vi "Update DAQ Parameters.vi"(8 "error in (no error)":errorcluster={"status"=FALSE, "code"=0, "source"="Abort\rATS : ApiSuccess (512)"}, 11 "DAQ Class in":refnum<class "DAQ Class.lvclass">=refnum) -> (0 "error out":errorcluster={"status"=FALSE, "code"=0, "source"="Abort\rATS : ApiSuccess (512)"}, 2 "DAQ Parameters Out":T1={"Points Per A-Scan"=1024, "A-Scans Per B-Scan"=250, "Number of B-Scans"=1, "A-Scans Per Transfer"=1, "Trigger Voltage"=0.0, "Trigger Source"=enum."External", "Trigger Slope"=enum."Rising", "Channel"=enum."Channel 1", "Clock"=enum."Internal Clock", "Bits per Sample"=0.0, "Range"=0.0}, 3 "DAQ Class out":refnum<class "DAQ Class.lvclass">)   [LabVIEW 2014, in "DAQ Class.lvclass"]
uses:
  DAQ Class.lvclass
  ATS660/ATS660 Class.lvclass
  DAQ Parameters.ctl
  Trigger Source.ctl
  Trigger Slope.ctl
  Type Defs/OCT DAQ Channel Data Type.ctl
  Clock Control.ctl
panel:
  in  "DAQ Parameters":T1={"Points Per A-Scan"=1280, "A-Scans Per B-Scan"=250, "Number of B-Scans"=1, "A-Scans Per Transfer"=250, "Trigger Voltage"=140.0, "Trigger Source"=enum."External", "Trigger Slope"=enum."Rising", "Channel"=enum."Channel 1", "Clock"=enum."External Clock", "Bits per Sample"=16.0, "Range"=4.0}
  in  "OK Button":bool
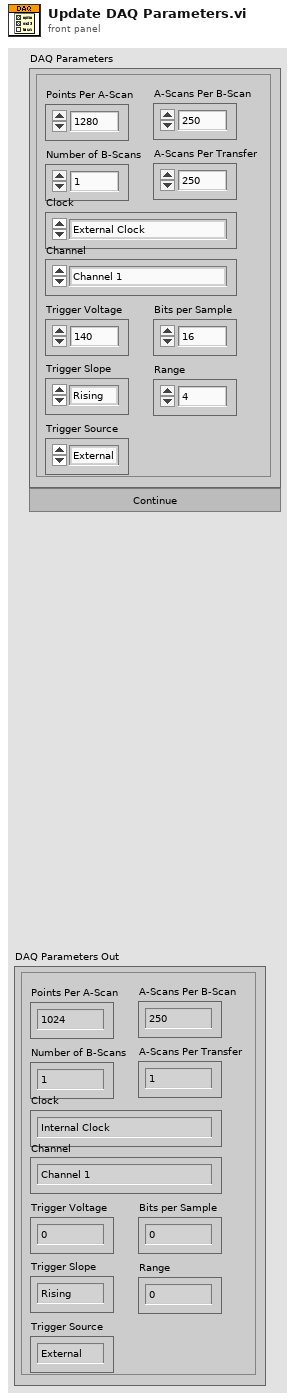
[diagram p1: front panel]
types:
  T1 = typedef "DAQ Class.lvclass/DAQ Parameters.ctl" = cluster{"Points Per A-Scan":u32, "A-Scans Per B-Scan":u32, "Number of B-Scans":u32, "A-Scans Per Transfer":u32, "Trigger Voltage":sgl, "Trigger Source":T2, "Trigger Slope":T3, "Channel":T4, "Clock":T5, "Bits per Sample":dbl, "Range":dbl}
  T2 = typedef "DAQ Class.lvclass/Trigger Source.ctl" = enum16{"External", "Channel A", "Channel B"}
  T3 = typedef "DAQ Class.lvclass/Trigger Slope.ctl" = enum16{"Rising", "Falling"}
  T4 = typedef "OCT DAQ Channel Data Type.ctl" = enum16{"Channel 1", "Channel 2", "Channel 1 and 2"}
  T5 = typedef "DAQ Class.lvclass/Clock Control.ctl" = enum16{"Internal Clock", "External Clock"}
  T6 = enum8{"Enabled", "Disabled", "Disabled and Grayed Out"}
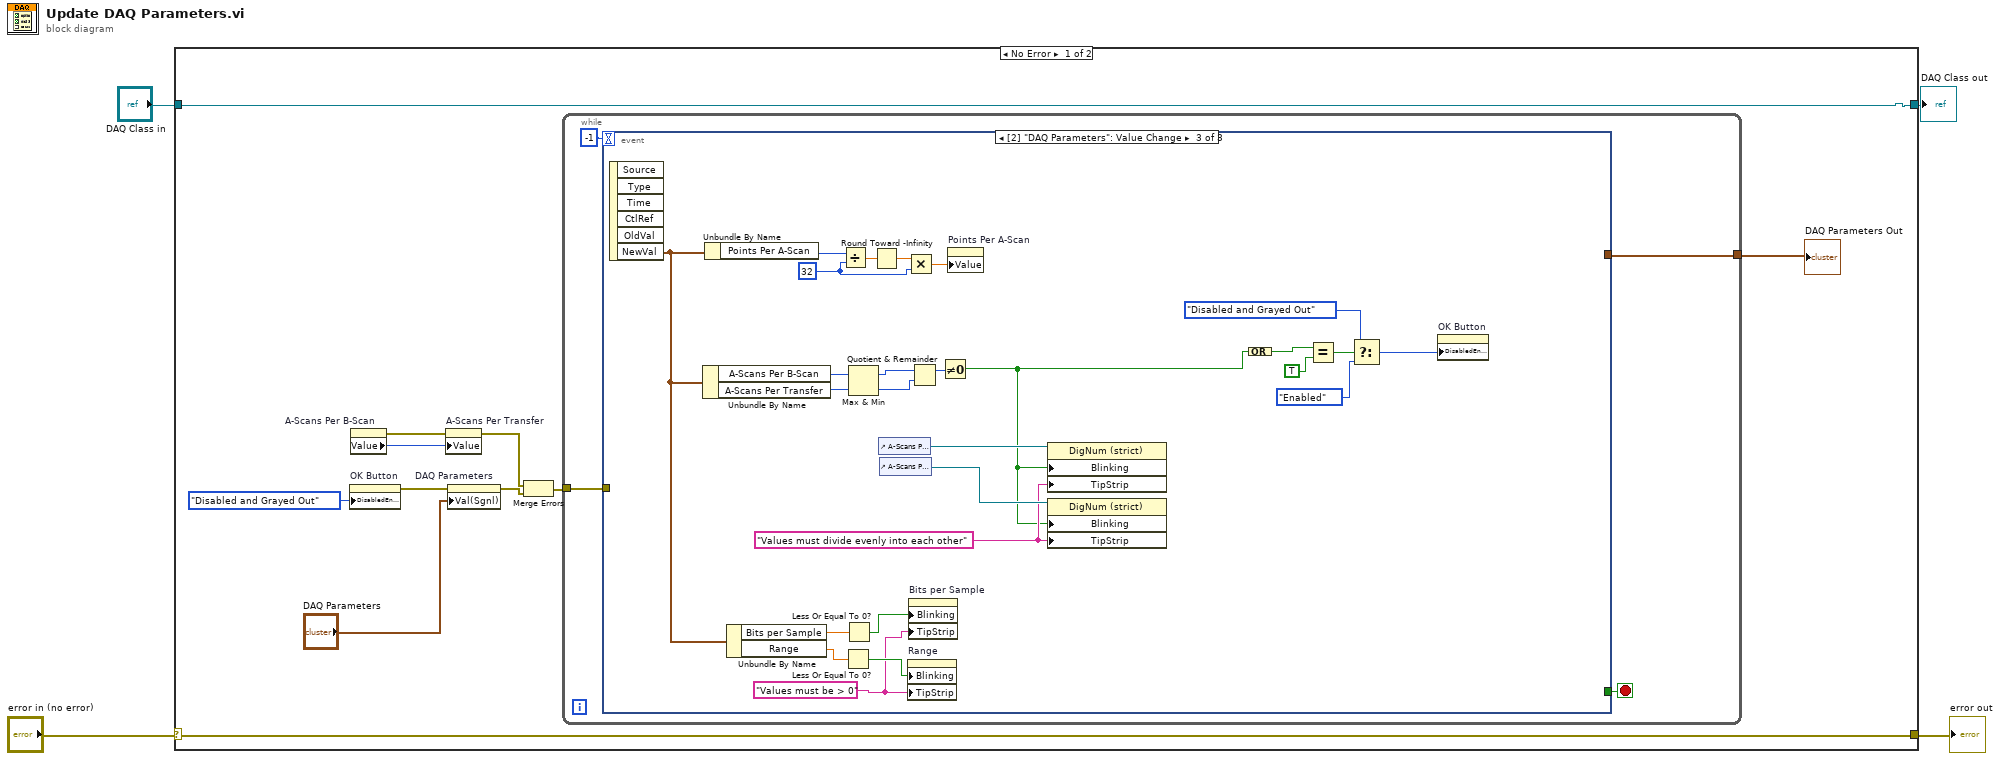
[diagram p0: block diagram]
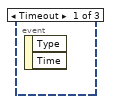
[diagram p2: hidden frame]
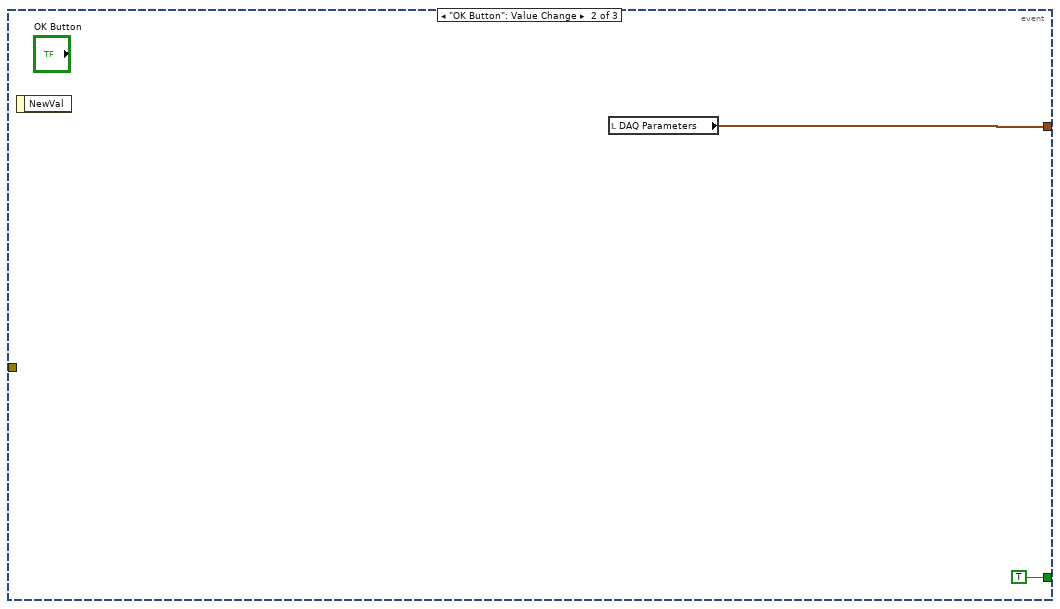
[diagram p3: hidden frame]
diagram:
  n1 = case shown="No Error" "error in (no error)" {
    selector: "error in (no error)" -> [w15 w49]
    tunnel: [w15 w49] -> w3
    tunnel: [w14 w48] -> w1
    tunnel: "DAQ Class in" -> [w14 w48]
    frame No Error {
      n2 = property on="OK Button" class="Bool"("DisabledEnum"=T6."Disabled and Grayed Out" ("Disabled")) -> (error out=w11:errorcluster)  [unwired: 2 in, 1 out]
      n3 = property on="A-Scans Per B-Scan" class="DigNum (strict)"() -> (error out=w10:errorcluster, "Value"=w9:u32)  [unwired: 2 in, 1 out]
      n4 = property on="A-Scans Per Transfer" class="DigNum (strict)"(error in=w10, "Value"=w9) -> (error out=w7:errorcluster)  [unwired: 1 in, 1 out]
      n5 = property on="DAQ Parameters" class="Clust (strict)"(error in=w11, "Val(Sgnl)"="DAQ Parameters") -> (error out=w8:errorcluster)  [unwired: 1 in, 1 out]
      n6 = Merge Errors(w7, w8) -> (w6:errorcluster)
      n7 = while {
        tunnel: [w17] -> w13
        tunnel: w6 -> [w16]
        stop <- w18 stop-if-true
        n8 = event shown="[2] \"DAQ Parameters\": Value Change" {
          selector: _ -> [_ _ _]
          dyn-events: _ -> [_ _ _]
          timeout: -1 -> [_ _ _]
          tunnel: [_ TRUE _] -> w18
          tunnel: [_ w20 _] -> w17
          tunnel: w16 -> [_ _ _]
          event Timeout {
            n9 = event-data() -> ()  [unwired: 1 in, 2 out]
          }
          event "OK Button": Value Change {
            n10 = event-data() -> ()  [unwired: 1 in, 1 out]
            n11 = local read "DAQ Parameters"() -> (w20:T1)
          }
          event Value Change {
            w27 = "Values must be > 0" ("Tip Strip")
            w44 = "Values must divide evenly into each other" ("Tip Strip")
            w23 = u32 32 ("y")
            n12 = event-data() -> ("NewVal"=w32:T1)  [unwired: 1 in, 5 out]
            n13 = Unbundle By Name(w32) -> ("A-Scans Per B-Scan"=w36:u32, "A-Scans Per Transfer"=w35:u32)
            n14 = Unbundle By Name(w32) -> ("Points Per A-Scan"=w26:u32)
            n15 = Unbundle By Name(w32) -> ("Bits per Sample"=w31:dbl, "Range"=w30:dbl)
            n16 = Divide(x=w26, y=w23) -> (x/y=w25:dbl)
            n17 = Less Or Equal To 0?(x=w30) -> (x <= 0?=w28:bool)
            n18 = Less Or Equal To 0?(x=w31) -> (x <= 0?=w29:bool)
            n19 = Max & Min(x=w36, y=w35) -> (max(x,y)=w34:u32, min(x,y)=w33:u32)
            n20 = Round Toward -Infinity(1:w25) -> (0:w24:dbl)
            n21 = control-ref of="A-Scans Per B-Scan"() -> (w46:refnum<vi>)
            n22 = control-ref of="A-Scans Per Transfer"() -> (w45:refnum<vi>)
            n23 = Multiply(x=w24, y=w23) -> (x*y=w22:dbl)
            n24 = property on="Range" class="DigNum (strict)"("Blinking"=w28, "TipStrip"=w27) -> ()  [unwired: 2 in, 2 out]
            n25 = property on="Bits per Sample" class="DigNum (strict)"("Blinking"=w29, "TipStrip"=w27) -> ()  [unwired: 2 in, 2 out]
            n26 = Quotient & Remainder(x=w34, y=w33) -> (x-y*floor(x/y)=w47:u32)  [unwired: 1 out]
            n27 = Not Equal To 0?(x=w47) -> (x != 0?=w37:bool)
            n28 = property on="Points Per A-Scan" class="DigNum (strict)"("Value"=w22) -> ()  [unwired: 2 in, 2 out]
            n29 = property class="DigNum (strict)"(reference=w46, "Blinking"=w37, "TipStrip"=w44) -> ()  [unwired: 1 in, 2 out]
            n30 = property class="DigNum (strict)"(reference=w45, "Blinking"=w37, "TipStrip"=w44) -> ()  [unwired: 1 in, 2 out]
            n31 = Compound Arithmetic op=OR(w37) -> (w43:bool)
            n32 = Equal?(x=w43, y=TRUE) -> (x = y?=w41:bool)
            n33 = Select(t=T6."Disabled and Grayed Out" ("Disabled"), s=w41, f=T6."Enabled" ("Disabled")) -> (s? t:f=w40:T6)
            n34 = property on="OK Button" class="Bool"("DisabledEnum"=w40) -> ()  [unwired: 2 in, 2 out]
          }
        }
      }
      "DAQ Parameters Out" <- w13
    }
    frame Error {
    }
  }
  "error out" <- w3
  "DAQ Class out" <- w1
